vi "CC Data Logging Loop.vi"(11 "user event":refnum<user-event>) -> ()   [LabVIEW 2024]
uses:
  hk-channel-class/hk-channel-class/HK Table/HK Table.lvclass
  Subsystems/SS cluster Data Queue type.ctl
  CC enum Current Values Action.ctl
  Subsystems/SS cluster New Image Data.ctl
  library/Activity Log/Activity Log enum Action .ctl
  typedefs/CC cluster Alarm Data.ctl
  typedefs/CC enum Alarm Action.ctl
  typedefs/CC cluster System Settings.ctl
  hk-channel-class/hk-channel-class/HK Item/HK Item.lvclass
panel:
  out "error out":errorcluster
  in  "error in (no error)":errorcluster
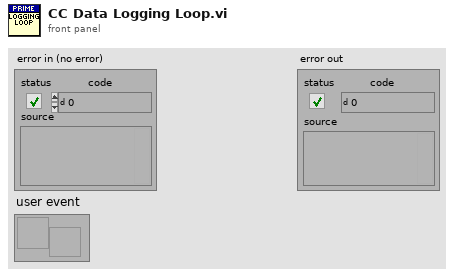
[diagram p1: front panel]
types:
  T1 = cluster{"HK Channels":refnum<class "HK Table.lvclass">, "Data Q":refnum<queue>, "user event":refnum<user-event>}
  T2 = typedef "CC enum Current Values Action.ctl" = enum16{"Init", "Write Item", "Write Array", "Read Item", "Read Array", "Read All", "Add Channels", "New File", "Add Message", "Get Current Values", "Close"}
  T3 = typedef "SS cluster New Image Data.ctl" = cluster{"Frame number":i32, "Detector #":u16, "FITS file":path, "File size":i64}
  T4 = typedef "Activity Log enum Action .ctl" = enum16{"Add Entry", "Get Log", "Restore From Disk", "Save to Disk", "Init", "Clear"}
  T5 = typedef "SS cluster Data Queue type.ctl" = cluster{"Source":string, "Type":string, "Data":variant}
  T6 = typedef "CC enum Alarm Action.ctl" = enum16{"Init", "Add Alarm", "Get Alarms", "Clear Alarm", "Clear All Alarms"}
  T7 = typedef "CC cluster Alarm Data.ctl" = cluster{"Measured Value":dbl, "Alarm Low":dbl, "Alarm High":dbl, "Message":string, "Source":string}
  T8 = typedef "CC cluster System Settings.ctl" = cluster{"HK Table Name":string, "Images Folder":path, "Obs File":path}
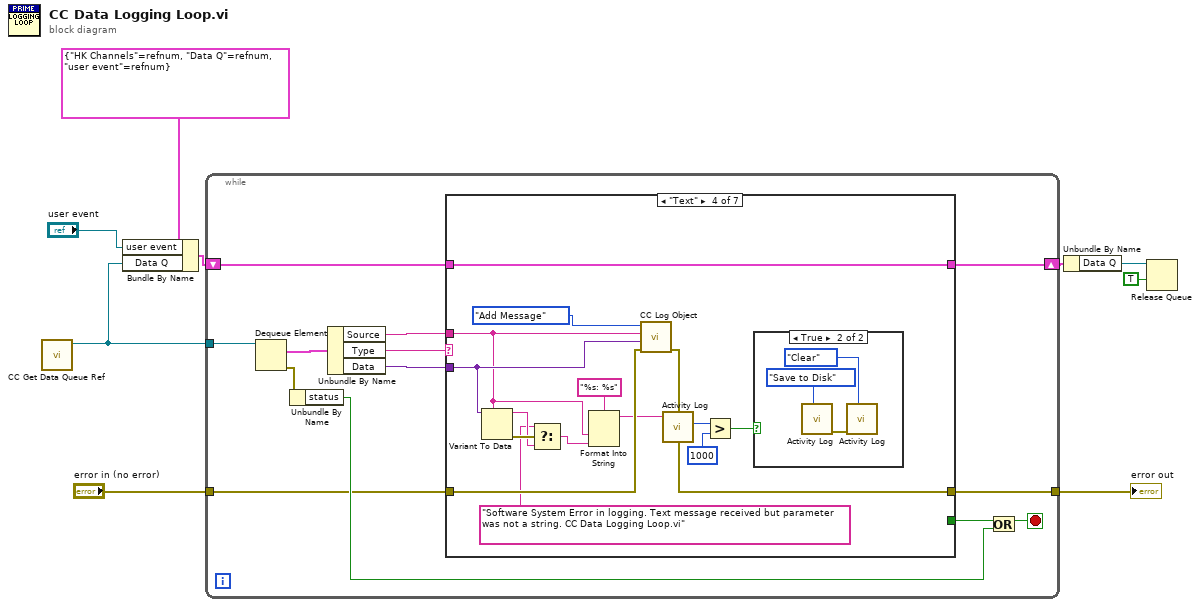
[diagram p0: block diagram]
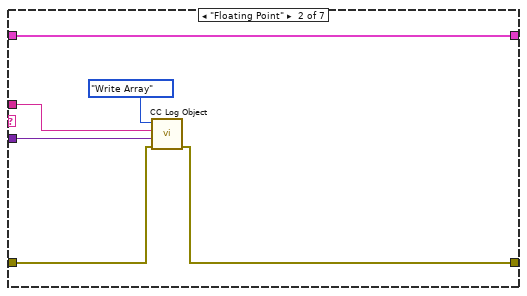
[diagram p3: hidden frame]
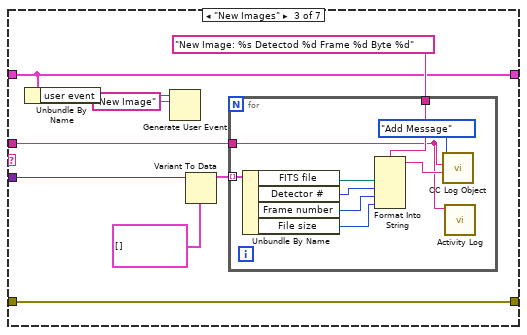
[diagram p4: hidden frame]
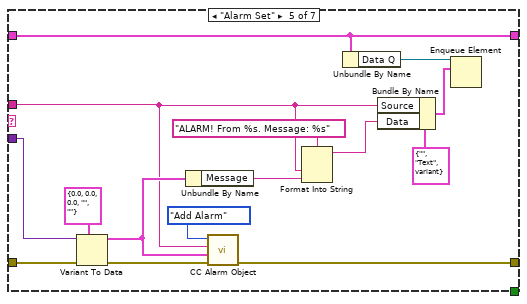
[diagram p6: hidden frame]
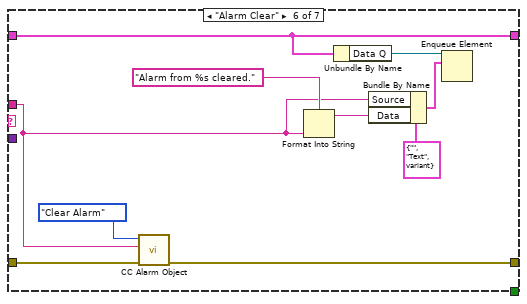
[diagram p7: hidden frame]
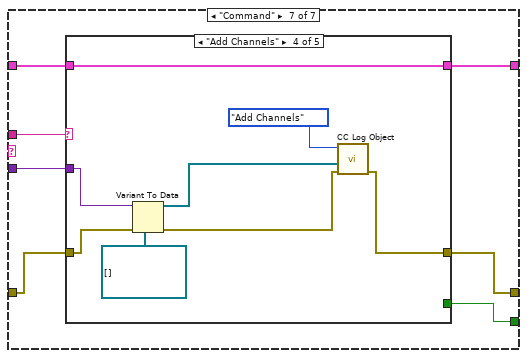
[diagram p8: hidden frame]
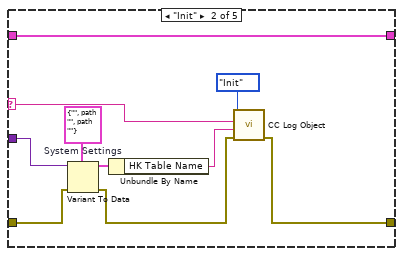
[diagram p10: hidden frame]
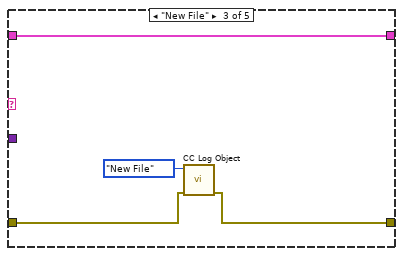
[diagram p11: hidden frame]
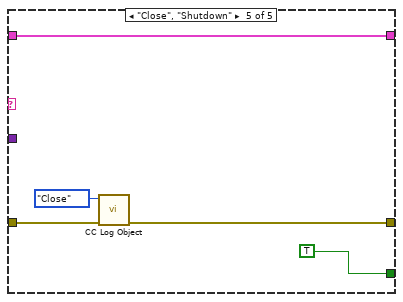
[diagram p12: hidden frame]
diagram:
  n1 = call "CC Get Data Queue Ref.vi"() -> ("Data Q"=w7:refnum<queue>)  [unwired: 10 in, 1 out]
  n2 = Bundle By Name(cluster=T1 {"HK Channels"=refnum, "Data Q"=refnum, "user event"=refnum}, "user event"="user event", "Data Q"=w7) -> (w5:T1)
  n3 = while {
    tunnel: w7 -> [w22]
    shift-right: [w12] -> w4
    shift-left: w5 -> [w16]
    tunnel: "error in (no error)" -> [w17]
    tunnel: [w11] -> w8
    stop <- w20 stop-if-true
    n4 = Dequeue Element(queue=w22) -> (element=w21:T5, error out=w19:errorcluster)  [unwired: 2 in, 2 out]
    n5 = Unbundle By Name(w19) -> ("status"=w18:bool)
    n6 = Unbundle By Name(w21) -> ("Source"=w14:string, "Type"=w15:string, "Data"=w13:variant)
    n7 = case shown="\"Text\"" w15 {
      tunnel: w13 -> [_ w28 w39 w59 w81 _ w95]
      tunnel: w16 -> [w24 w27 w33 w62 w75 w83 w98]
      tunnel: [w24 w27 w33 w62 w75 w83 w97] -> w12
      tunnel: w14 -> [_ w29 w35 w57 w69 w82 w92]
      tunnel: w17 -> [w23 w26 w34 w61 w78 w89 w96]
      tunnel: [w23 w25 w34 w60 w76 w90 w94] -> w11
      tunnel: [_ _ _ _ _ _ w93] -> w10
      frame "False", Default {
      }
      frame "Floating Point" {
        n8 = call "CC Log Object.vi"("error in (no error)"=w26, "Data"=w28, "Source"=w29, "Action"=CC_enum_Current_Values_Action."Write Array") -> ("error out"=w25:errorcluster)  [unwired: 5 in, 2 out]
      }
      frame "New Images" {
        n9 = Unbundle By Name(w33) -> ("user event"=w32:refnum<user-event>)
        n10 = Generate User Event(user event=w32, event data cluster="New Image" ("event data")) -> ()  [unwired: 2 in, 2 out]
        n11 = Variant To Data(type=T3[] [], Variant=w39) -> (data=w37:T3[])  [unwired: 1 in, 1 out]
        n12 = for {
          tunnel: w37 -> [w48] mode=indexing
          tunnel: "New Image: %s Detectod %d Frame %d Byte %d" ("format string") -> [w47]
          tunnel: w35 -> [w40]
          n13 = Unbundle By Name(w48) -> ("FITS file"=w46:path, "Detector #"=w45:u16, "Frame number"=w44:i32, "File size"=w43:i64)
          n14 = Format Into String(format string=w47, w46, w45, w44, w43) -> (resulting string=w41:string)  [unwired: 2 in, 1 out]
          n15 = call "CC Log Object.vi"("Data"=w41, "Source"=w40, "Action"=CC_enum_Current_Values_Action."Add Message") -> ()  [unwired: 6 in, 3 out]
          n16 = call "Activity Log.vi"("Message Log Entry"=w40) -> ()  [unwired: 8 in, 3 out]
        }
      }
      frame "Text" {
        n17 = Variant To Data(type=w57, Variant=w59) -> (data=w54:string, error out=w55:errorcluster)  [unwired: 1 in]
        n18 = Select(t="Software System Error in logging. Text message received but parameter was not a string. CC Data Logging Loop.vi", s=w55, f=w54) -> (s? t:f=w53:string)
        n19 = Format Into String(format string="%s: %s", w57, w53) -> (resulting string=w56:string)  [unwired: 2 in, 1 out]
        n20 = call "CC Log Object.vi"("error in (no error)"=w61, "Data"=w59, "Source"=w57, "Action"=CC_enum_Current_Values_Action."Add Message") -> ("error out"=w60:errorcluster)  [unwired: 5 in, 2 out]
        n21 = call "Activity Log.vi"("Message Log Entry"=w56) -> ("rows"=w51:i32)  [unwired: 8 in, 2 out]
        n22 = Greater?(x=w51, y=1000) -> (0:w49:bool)
        n23 = case shown="True" w49 {
          frame False {
          }
          frame True {
            n24 = call "Activity Log.vi"("Action"=Activity_Log_enum_Action_."Save to Disk") -> ("Error Out"=w65:errorcluster)  [unwired: 8 in, 2 out]
            n25 = call "Activity Log.vi"("Action"=Activity_Log_enum_Action_."Clear", "Error In"=w65) -> ()  [unwired: 7 in, 3 out]
          }
        }
      }
      frame "Alarm Set" {
        n26 = Variant To Data(error in=w78, type=T7 {"Measured Value"=0.0, "Alarm Low"=0.0, "Alarm High"=0.0, "Message"="", "Source"=""}, Variant=w81) -> (data=w72:T7, error out=w77:errorcluster)
        n27 = Unbundle By Name(w72) -> ("Message"=w68:string)
        n28 = call "CC Alarm Object.vi"("error in (no error)"=w77, "Alarm"=w72, "Source"=w69, "Alarm Action"=CC_enum_Alarm_Action."Add Alarm") -> ("error out"=w76:errorcluster)  [unwired: 5 in, 2 out]
        n29 = Format Into String(format string="ALARM! From %s. Message: %s", w69, w68) -> (resulting string=w67:string)  [unwired: 2 in, 1 out]
        n30 = Unbundle By Name(w75) -> ("Data Q"=w74:refnum<queue>)
        n31 = Bundle By Name(cluster=T5 {"Source"="", "Type"="Text", "Data"=variant} ("element"), "Source"=w69, "Data"=w67) -> (w71:T5)
        n32 = Enqueue Element(queue=w74, element=w71) -> ()  [unwired: 2 in, 3 out]
      }
      frame "Alarm Clear" {
        n33 = call "CC Alarm Object.vi"("error in (no error)"=w89, "Source"=w82, "Alarm Action"=CC_enum_Alarm_Action."Clear Alarm") -> ("error out"=w90:errorcluster)  [unwired: 6 in, 2 out]
        n34 = Format Into String(format string="Alarm from %s cleared.", w82) -> (resulting string=w84:string)  [unwired: 2 in, 1 out]
        n35 = Unbundle By Name(w83) -> ("Data Q"=w88:refnum<queue>)
        n36 = Bundle By Name(cluster=T5 {"Source"="", "Type"="Text", "Data"=variant} ("element"), "Source"=w82, "Data"=w84) -> (w86:T5)
        n37 = Enqueue Element(queue=w88, element=w86) -> ()  [unwired: 2 in, 3 out]
      }
      frame "Command" {
        n38 = case shown="\"Add Channels\"" w92 {
          selector: w92 -> [_ w107 _ _ _]
          tunnel: w98 -> [w99 w105 w114 w119 w127]
          tunnel: [w99 w105 w114 w119 w127] -> w97
          tunnel: w96 -> [w100 w101 w111 w117 w125]
          tunnel: [w100 w104 w112 w116 w124] -> w94
          tunnel: [_ _ _ _ TRUE] -> w93
          tunnel: w95 -> [_ w103 _ w115 _]
          frame "False", Default {
          }
          frame "Init" {
            w110 = T8 {"HK Table Name"="", "Images Folder"=path "", "Obs File"=path ""}  # System Settings
            n39 = Variant To Data(error in=w101, type=w110, Variant=w103) -> (data=w109:T8, error out=w102:errorcluster)
            n40 = Unbundle By Name(w109) -> ("HK Table Name"=w106:string)
            n41 = call "CC Log Object.vi"("error in (no error)"=w102, "Data"=w106, "Source"=w107, "Action"=CC_enum_Current_Values_Action."Init") -> ("error out"=w104:errorcluster)  [unwired: 5 in, 2 out]
          }
          frame "New File" {
            n42 = call "CC Log Object.vi"("error in (no error)"=w111, "Action"=CC_enum_Current_Values_Action."New File") -> ("error out"=w112:errorcluster)  [unwired: 7 in, 2 out]
          }
          frame "Add Channels" {
            n43 = Variant To Data(error in=w117, type=refnum<class "HK Item.lvclass">[] [], Variant=w115) -> (data=w120:refnum<class "HK Item.lvclass">[], error out=w118:errorcluster)
            n44 = call "CC Log Object.vi"("error in (no error)"=w118, "Data"=w120, "Action"=CC_enum_Current_Values_Action."Add Channels") -> ("error out"=w116:errorcluster)  [unwired: 6 in, 2 out]
          }
          frame "Close", "Shutdown" {
            n45 = call "CC Log Object.vi"("error in (no error)"=w125, "Action"=CC_enum_Current_Values_Action."Close") -> ("error out"=w124:errorcluster)  [unwired: 7 in, 2 out]
          }
        }
      }
    }
    n46 = Or(x=w10, y=w18) -> (x .or. y?=w20:bool)
  }
  "error out" <- w8
  n47 = Unbundle By Name(w4) -> ("Data Q"=w3:refnum<queue>)
  n48 = Release Queue(queue=w3, force destroy? (F)=TRUE) -> ()  [unwired: 1 in, 3 out]
